vi "Get frame rate.vi"(8 "error in (no error)":errorcluster, 11 "DAQOrcaFlash in":refnum<class "DAQOrcaFlash.lvclass">) -> (0 "error out":errorcluster, 3 "DAQOrcaFlash out":refnum<class "DAQOrcaFlash.lvclass">)   [LabVIEW 2012, in "DAQOrcaFlash.lvclass"]
uses:
  DAQOrcaFlash.lvclass
  DAQOrcaFlash.lvclass/DAQOrcaFlash.ctl
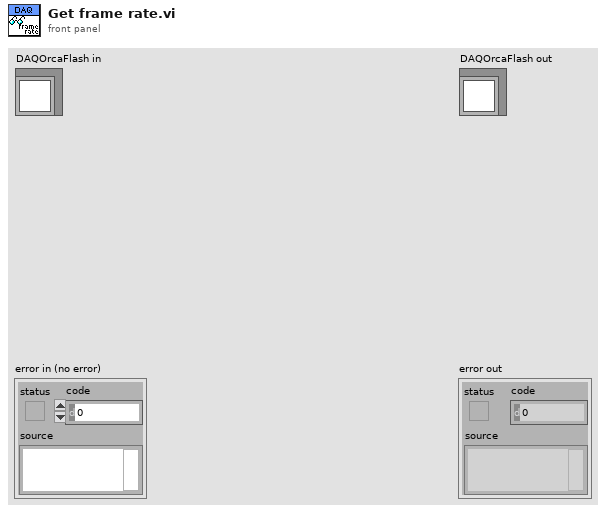
[diagram p1: front panel]
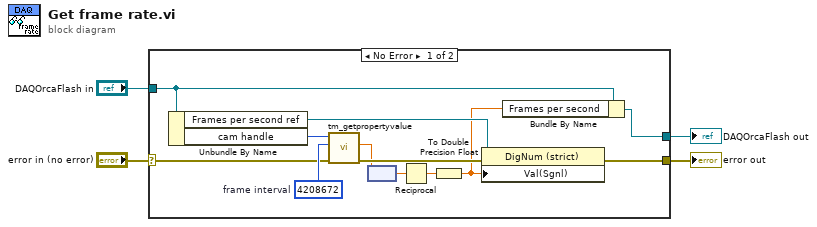
[diagram p0: block diagram]
diagram:
  n1 = case shown="No Error" "error in (no error)" {
    selector: "error in (no error)" -> [w13 w18]
    tunnel: [w5 w18] -> w3
    tunnel: [w6 w17] -> w1
    tunnel: "DAQOrcaFlash in" -> [w16 w17]
    frame No Error {
      w14 = u32 4208672  # frame interval
      n2 = Unbundle By Name(w16) -> ("Frames per second ref"=w15:refnum<vi>, "cam handle"=w12:u32)
      n3 = call <userlib>:"tm_getpropertyvalue.vi"("error in (no error)"=w13, "Property ID"=w14, "Handle in"=w12) -> ("error out"=w11:errorcluster, "Value in"=w10:sgl)  [unwired: 6 in, 1 out]
      n4 = node(w10) -> (w9:sgl[unit])
      n5 = Reciprocal(x=w9) -> (1/x=w8:sgl[unit])
      n6 = To Double Precision Float(number=w8) -> (double precision float=w7:dbl[unit])
      n7 = property class="DigNum (strict)"(reference=w15, error in=w11, "Val(Sgnl)"=w7) -> (error out=w5:errorcluster)  [unwired: 1 out]
      n8 = Bundle By Name(cluster=w16, "Frames per second"=w7) -> (w6:refnum<class "DAQOrcaFlash.lvclass">)
    }
    frame Error {
    }
  }
  "error out" <- w3
  "DAQOrcaFlash out" <- w1
